vi "dataProcess_spectrMax.vi"(2 "spectr const":sgl[](array[numeric]) format="%.2f", 4 "spectr":sgl[](array[numeric]) format="%.2f", 5 "error in (no error)":errorcluster) -> (18 "spectr max":sgl[](array[numeric]) format="%.2f", 19 "error out":errorcluster)   [LabVIEW 2010, in "OSA.lvclass"]
doc: "This calculates each data point in spectr as the maximum of spectr and the same data point in spectr const. \n\nParameters\n\nspectr: on successful return the maximum of spectr and spectr const, point by point \n\nspectr const: the spectrum to compare with. \n\nlength: length of the data arrays spectr and spectr const."
uses:
  OSA.lvclass
  FTSLib.dll
panel:
  in  "length":u32
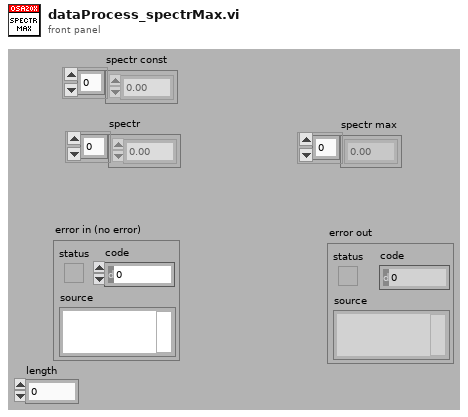
[diagram p1: front panel]
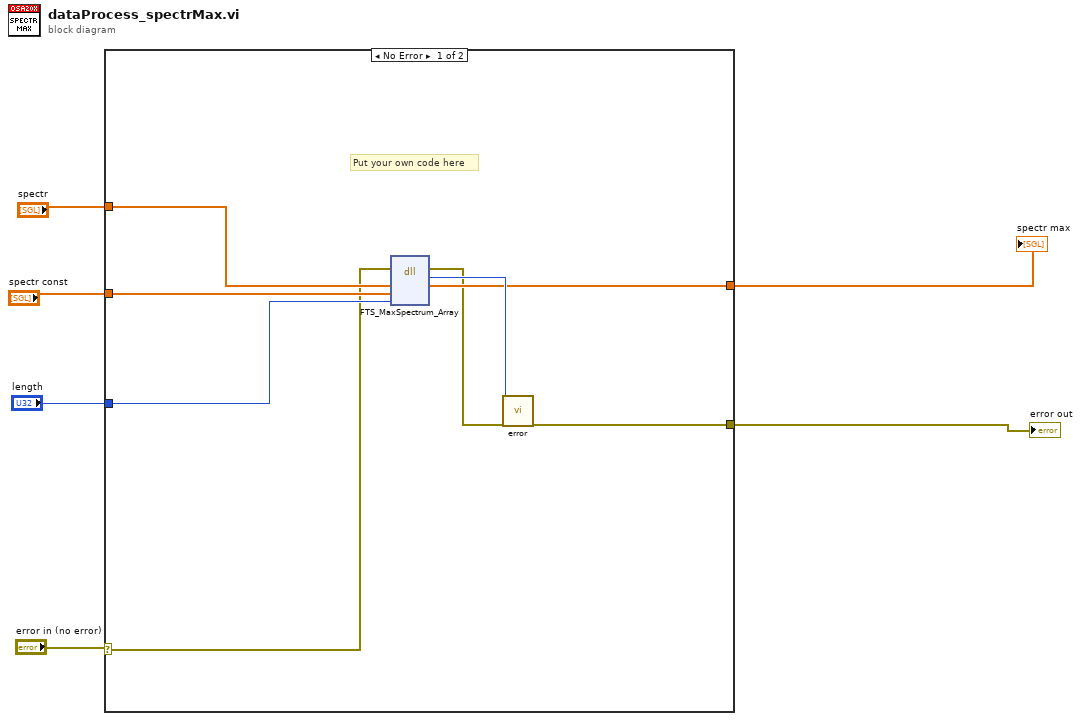
[diagram p0: block diagram]
diagram:
  n1 = case shown="No Error" "error in (no error)" {
    selector: "error in (no error)" -> [w8 w16]
    tunnel: [w13 w16] -> w6
    tunnel: "spectr const" -> [w12 _]
    tunnel: "spectr" -> [w11 w15]
    tunnel: "length" -> [w10 _]
    tunnel: [w9 w15] -> w1
    frame No Error {
      # "Put your own code here"
      n2 = dll-call lib="FTSLib.dll" fn="FTS_MaxSpectrum_Array"(error in=w8, "spectrum_1"=w11, "spectrum_2"=w12, "length"=w10) -> (error out=w7:errorcluster, "return type"=w14:i32, "spectrum_1"=w9:sgl[])  [unwired: 4 in, 1 out]
      n3 = call "error.vi"("result code"=w14, "error in (no error)"=w7) -> ("error out"=w13:errorcluster)  [unwired: 15 in, 2 out]
    }
    frame Error {
      # "Error"
    }
  }
  "error out" <- w6
  "spectr max" <- w1
